vi "porownanie algorytmow histogramow.vi"() -> ()   [LabVIEW 2013]
panel:
  out "Czas algorytmu 3":u32
  out "Histogram 3":i32[](graph)
  out "Przedziały (min; max) 3":dbl[][](array[numeric])
  out "Czas algorytmu 2":u32
  out "Histogram 2":i32[](graph)
  out "Przedziały (min; max) 2":dbl[][](array[numeric])
  out "Czas algorytmu 1":u32
  out "Przedziały (min; max)":dbl[][](array[numeric])
  out "Histogram":i32[](graph)
  in  "Liczba przedziałów":i32
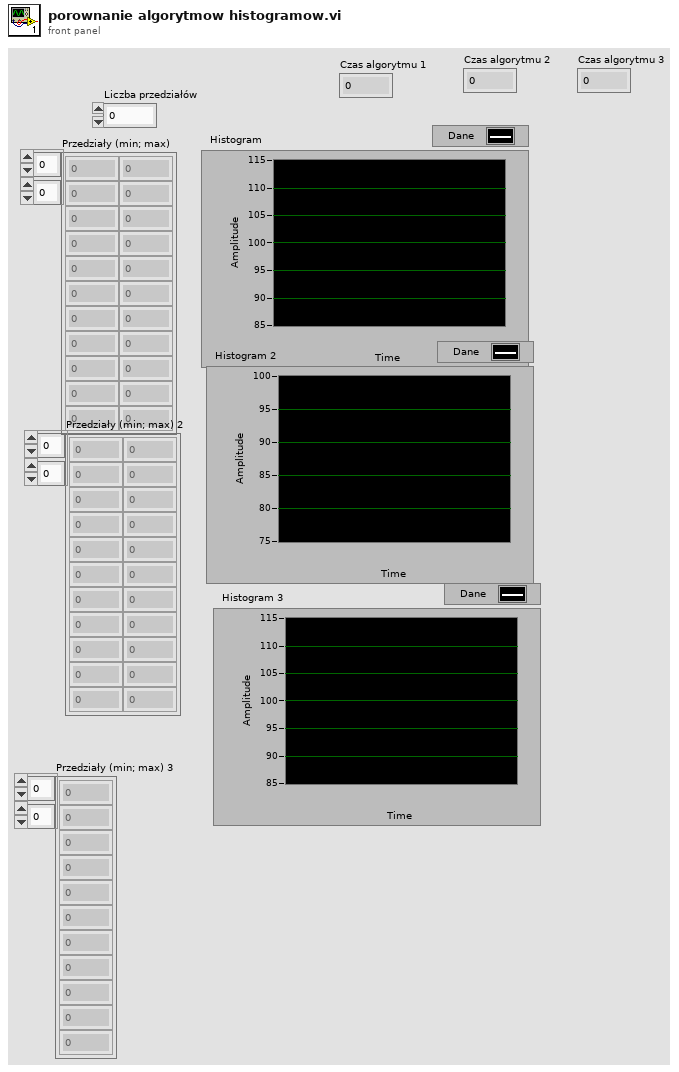
[diagram p1: front panel]
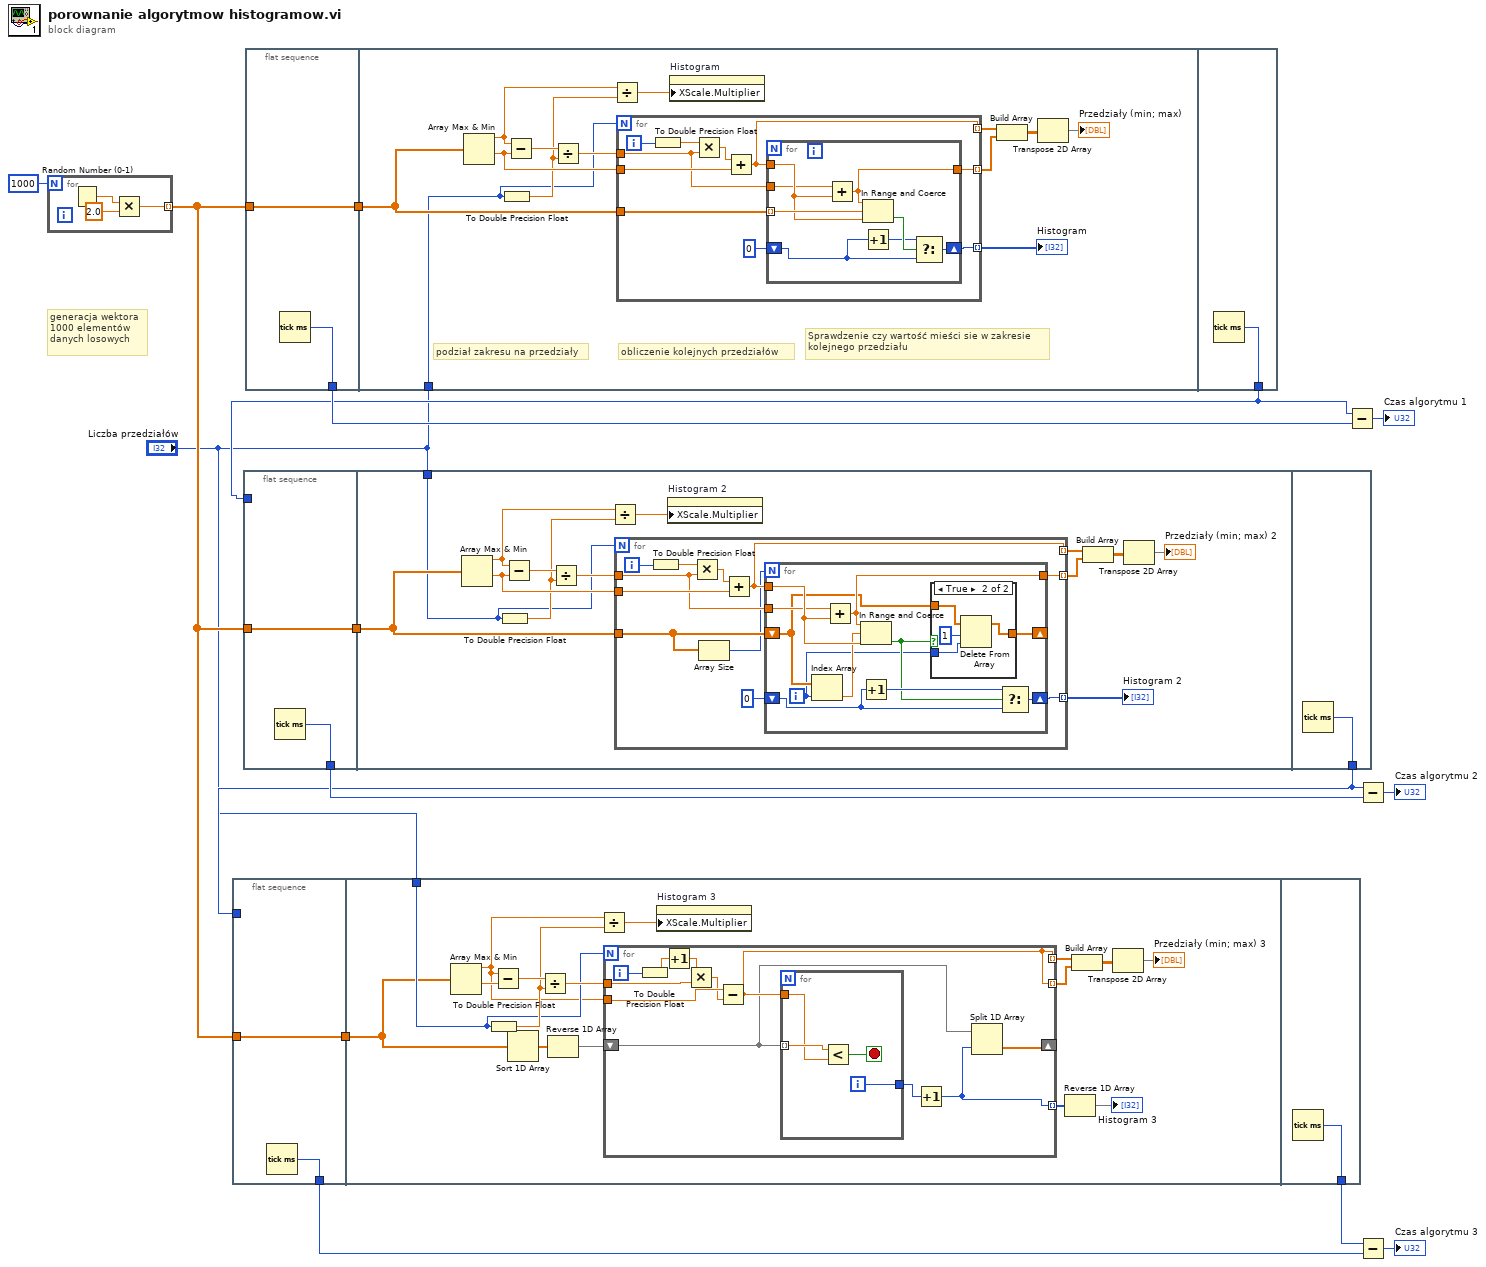
[diagram p0: block diagram]
diagram:
  # "generacja wektora\n1000 elementów\ndanych losowych"
  n1 = for {
    N: 1000 -> [_]
    tunnel: [w16] -> w2 mode=indexing
    n2 = Random Number (0-1)() -> (number: 0 to 1=w18:dbl)
    n3 = Multiply(x=w18, y=2.0) -> (x*y=w16:dbl)
  }
  n4 = flat-sequence {
    tunnel: w2 -> [w20]
    tunnel: [w20] -> w7
    tunnel: [w19] -> w4
    tunnel: w3 -> [_]
    tunnel: w7 -> [w26]
    tunnel: "Liczba przedziałów" -> [w27]
    tunnel: [w52] -> w5
    frame #0 {
      n5 = Tick Count (ms)() -> (millisecond timer value=w19:u32)
    }
    frame #1 {
      n6 = Array Max & Min(array=w26) -> (max value=w25:dbl, min value=w34:dbl)  [unwired: 2 out]
      n7 = To Double Precision Float(number=w27) -> (double precision float=w28:dbl)
      n8 = Subtract(x=w25, y=w34) -> (x-y=w36:dbl)
      n9 = Sort 1D Array(array=w26) -> (sorted array=w23:dbl[])
      n10 = Divide(x=w36, y=w28) -> (x/y=w35:dbl)
      n11 = Reverse 1D Array(array=w23) -> (reversed array=w24:dbl[])
      n12 = Divide(x=w25, y=w28) -> (x/y=w33:dbl)
      n13 = for {
        N: w27 -> [_]
        tunnel: w35 -> [w46]
        tunnel: w25 -> [w45]
        tunnel: [w37] -> w22 mode=indexing
        tunnel: [w43] -> w32 mode=indexing
        tunnel: [w43] -> w31 mode=indexing
        shift-right: [w38] -> _
        shift-left: w24 -> [w39]
        i -> [w47]
        n14 = To Double Precision Float(number=w47) -> (double precision float=w42:dbl)
        n15 = Increment(x=w42) -> (x+1=w41:dbl)
        n16 = Multiply(x=w41, y=w46) -> (x*y=w44:dbl)
        n17 = Subtract(x=w45, y=w44) -> (x-y=w43:dbl)
        n18 = for {
          tunnel: w39 -> [w51] mode=indexing
          tunnel: w43 -> [w50]
          tunnel: [w48] -> w40
          i -> [w48]
          stop <- w49 stop-if-true
          n19 = Less?(x=w51, y=w50) -> (x < y?=w49:bool)
        }
        n20 = Increment(x=w40) -> (x+1=w37:i32)
        n21 = Split 1D Array(array=w39, index=w37) -> (second subarray=w38:dbl[])  [unwired: 1 out]
      }
      n22 = property on="Histogram 3" class="WFGraph (strict)"("XScale.Multiplier"=w33) -> ()  [unwired: 2 in, 2 out]
      n23 = Reverse 1D Array(array=w22) -> (reversed array=→"Histogram 3":i32[])
      n24 = Build Array(w32, w31) -> (w29:dbl[][])
      n25 = Transpose 2D Array(2D array=w29) -> (transposed array=→"Przedziały (min; max) 3":dbl[][])
    }
    frame #2 {
      n26 = Tick Count (ms)() -> (millisecond timer value=w52:u32)
    }
  }
  n27 = flat-sequence {
    tunnel: w2 -> [w54]
    tunnel: [w54] -> w11
    tunnel: [w53] -> w9
    tunnel: w8 -> [_]
    tunnel: w11 -> [w66]
    tunnel: "Liczba przedziałów" -> [w55]
    tunnel: [w95] -> w3
    frame #0 {
      n28 = Tick Count (ms)() -> (millisecond timer value=w53:u32)
    }
    frame #1 {
      n29 = Array Max & Min(array=w66) -> (max value=w62:dbl, min value=w64:dbl)  [unwired: 2 out]
      n30 = To Double Precision Float(number=w55) -> (double precision float=w56:dbl)
      n31 = Subtract(x=w62, y=w64) -> (x-y=w67:dbl)
      n32 = Divide(x=w67, y=w56) -> (x/y=w65:dbl)
      n33 = Divide(x=w62, y=w56) -> (x/y=w61:dbl)
      n34 = for {
        N: w55 -> [_]
        tunnel: w66 -> [w69]
        tunnel: w65 -> [w72]
        tunnel: w64 -> [w77]
        tunnel: [w73] -> w63 mode=indexing
        tunnel: [w71] -> w60 mode=indexing
        tunnel: [w70] -> w59 mode=indexing
        i -> [w78]
        n35 = To Double Precision Float(number=w78) -> (double precision float=w76:dbl)
        n36 = Multiply(x=w76, y=w72) -> (x*y=w75:dbl)
        n37 = Array Size(array=w69) -> (size(s)=w68:i32)
        n38 = Add(x=w75, y=w77) -> (x+y=w71:dbl)
        n39 = for {
          N: w68 -> [_]
          tunnel: w71 -> [w86]
          shift-right: [w87] -> w73
          shift-left: 0 -> [w89]
          tunnel: w72 -> [w85]
          tunnel: [w84] -> w70
          shift-right: [w80] -> _
          shift-left: w69 -> [w81]
          i -> [w79]
          n40 = Index Array(array=w81, index=w79) -> (element=w83:dbl)
          n41 = Add(x=w85, y=w86) -> (x+y=w84:dbl)
          n42 = In Range and Coerce(upper limit=w84, x=w83, lower limit=w86) -> (In Range?=w82:bool)  [unwired: 1 out]
          n43 = Increment(x=w89) -> (x+1=w88:i32)
          n44 = case shown="True" w82 {
            tunnel: w81 -> [w90 w93]
            tunnel: [w90 w94] -> w80
            tunnel: w79 -> [_ w92]
            frame False {
            }
            frame True {
              n45 = Delete From Array(array=w93, length=1, index=w92) -> (array with subset deleted=w94:dbl[])  [unwired: 1 out]
            }
          }
          n46 = Select(t=w88, s=w82, f=w89) -> (s? t:f=w87:i32)
        }
      }
      "Histogram 2" <- w63
      n47 = property on="Histogram 2" class="WFGraph (strict)"("XScale.Multiplier"=w61) -> ()  [unwired: 2 in, 2 out]
      n48 = Build Array(w60, w59) -> (w57:dbl[][])
      n49 = Transpose 2D Array(2D array=w57) -> (transposed array=→"Przedziały (min; max) 2":dbl[][])
    }
    frame #2 {
      n50 = Tick Count (ms)() -> (millisecond timer value=w95:u32)
    }
  }
  n51 = flat-sequence {
    tunnel: w2 -> [w97]
    tunnel: [w97] -> w14
    tunnel: [w96] -> w13
    tunnel: w14 -> [w109]
    tunnel: "Liczba przedziałów" -> [w98]
    tunnel: [w129] -> w8
    frame #0 {
      n52 = Tick Count (ms)() -> (millisecond timer value=w96:u32)
    }
    frame #1 {
      # "Sprawdzenie czy wartość mieści sie w zakresie\nkolejnego przedziału"
      # "podział zakresu na przedziały"
      # "obliczenie kolejnych przedziałów"
      n53 = Array Max & Min(array=w109) -> (max value=w105:dbl, min value=w107:dbl)  [unwired: 2 out]
      n54 = To Double Precision Float(number=w98) -> (double precision float=w99:dbl)
      n55 = Subtract(x=w105, y=w107) -> (x-y=w110:dbl)
      n56 = Divide(x=w110, y=w99) -> (x/y=w108:dbl)
      n57 = Divide(x=w105, y=w99) -> (x/y=w104:dbl)
      n58 = for {
        N: w98 -> [_]
        tunnel: w109 -> [w119]
        tunnel: w108 -> [w113]
        tunnel: w107 -> [w118]
        tunnel: [w114] -> w106 mode=indexing
        tunnel: [w112] -> w103 mode=indexing
        tunnel: [w111] -> w102 mode=indexing
        i -> [w120]
        n59 = To Double Precision Float(number=w120) -> (double precision float=w117:dbl)
        n60 = Multiply(x=w117, y=w113) -> (x*y=w116:dbl)
        n61 = Add(x=w116, y=w118) -> (x+y=w112:dbl)
        n62 = for {
          tunnel: w119 -> [w128] mode=indexing
          tunnel: w112 -> [w123]
          shift-right: [w124] -> w114
          shift-left: 0 -> [w126]
          tunnel: w113 -> [w122]
          tunnel: [w121] -> w111
          n63 = Add(x=w122, y=w123) -> (x+y=w121:dbl)
          n64 = In Range and Coerce(upper limit=w121, x=w128, lower limit=w123) -> (In Range?=w127:bool)  [unwired: 1 out]
          n65 = Increment(x=w126) -> (x+1=w125:i32)
          n66 = Select(t=w125, s=w127, f=w126) -> (s? t:f=w124:i32)
        }
      }
      "Histogram" <- w106
      n67 = property on="Histogram" class="WFGraph (strict)"("XScale.Multiplier"=w104) -> ()  [unwired: 2 in, 2 out]
      n68 = Build Array(w103, w102) -> (w100:dbl[][])
      n69 = Transpose 2D Array(2D array=w100) -> (transposed array=→"Przedziały (min; max)":dbl[][])
    }
    frame #2 {
      n70 = Tick Count (ms)() -> (millisecond timer value=w129:u32)
    }
  }
  n71 = Subtract(x=w8, y=w13) -> (x-y=→"Czas algorytmu 1":u32)
  n72 = Subtract(x=w3, y=w9) -> (x-y=→"Czas algorytmu 2":u32)
  n73 = Subtract(x=w5, y=w4) -> (x-y=→"Czas algorytmu 3":u32)
